vi "fgt set session Pressure Unit.vi"(8 "error in (no error)":errorcluster, 11 "unit":T1) -> (0 "error out":errorcluster)   [LabVIEW 2020, in "fgt_SDK.lvlib"]
doc: "Set pressure unit for all initialized channels, default value is \"mbar\". If type is invalid an error is returned.\nEvery pressure read value and sent command will then use this unit.\nExample of type: \"mbar\", \"millibar\", \"kPa\" ..."
uses:
  fgt_SDK.lvlib
  TypeDefs/fgt_PRESSURE_UNIT.ctl
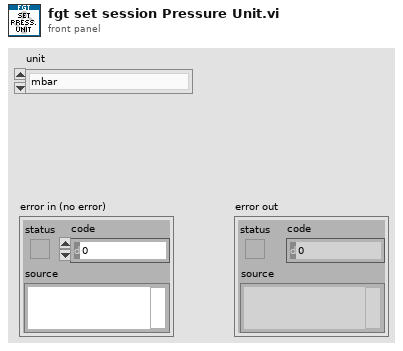
[diagram p1: front panel]
types:
  T1 = typedef "fgt_SDK.lvlib/fgt_PRESSURE_UNIT.ctl" = enum16{"mbar", "kPa", "PSI"}
  T2 = typedef "fgt_SDK.lvlib/fgt_STATUS_INFO.ctl" = cluster{"InstrType":T3, "instrSN":u16, "errorCode":u8, "infoCode":u8, "detail":string}
  T3 = typedef "fgt_SDK.lvlib/fgt_INSTRUMENT_TYPE.ctl" = enum32{"None", "MFCS", "MFCS_EZ", "FRP", "LineUP", "IPS"}
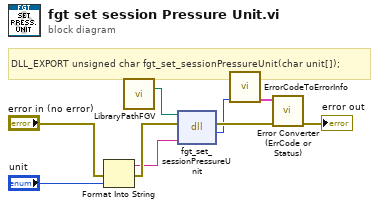
[diagram p0: block diagram]
diagram:
  # "DLL_EXPORT unsigned char fgt_set_sessionPressureUnit(char unit[]);"
  n1 = Format Into String(error in="error in (no error)", "unit") -> (resulting string=w4:string, error out=w5:errorcluster)  [unwired: 2 in]
  n2 = call "LibraryPathFGV.vi"() -> ("Path Out"=w1:path)  [unwired: 14 in, 1 out]
  n3 = dll-call lib="C:/Workspace/fgt-SDK/LabVIEW/dlls/fgt_SDK_*.*" fn="fgt_set_sessionPressureUnit"(path in=w1, error in=w5, "unit"=w4) -> (error out=w9:errorcluster, "return type"=w3:u8)  [unwired: 2 in, 1 out]
  n4 = call "ErrorCodeToErrorInfo.vi"("return type"=w3) -> ("StatusInfo"=w2:T2)  [unwired: 10 in]
  n5 = call "Error Converter (ErrCode or Status).vi"("error in (no error)"=w9, "StatusInfo"=w2) -> ("error out"=→"error out":errorcluster)  [unwired: 9 in]
